vi "Write I64.vi"(8 "error in (no error)":errorcluster, 9 "Timeout (ms)":i32, 10 "Data":i64, 11 "CIFTag in":refnum<class "CIF_CIPC_Chn_I64.lvclass">) -> (0 "error out":errorcluster, 1 "timed out?":bool, 3 "CIFTag out":refnum<class "CIF_CIPC_Chn_I64.lvclass">)   [LabVIEW 2021, in "CIF_CIPC_Chn_I64.lvclass"]
uses:
  CIF_CIPC_Chn_I64.lvclass
  D:/dev/Packages/CIF_Channels_Core/src/CIFChannels/CIFChannels.lvclass
  D:/dev/Packages/CIF_Channels_Core/src/CIPC_Channels/CIF_CIPC_Chan/CIF_CIPC_Chn.lvclass
  CIFChannels/CIFChannels.lvclass/CIFChannels.ctl
  CIF_CIPC_Chan/CIF_CIPC_Chn.lvclass/CIF_CIPC_Chn.ctl
  CIF_CIPC_Chn_I64.lvclass/CIF_CIPC_Chn_I64.ctl
  CIF_CIPC_Chan/Accessors/Read CIPC Channel.vi
  Write I64 Direct.vi/4dec1408-e4ff-48ac-a735-b713bf84484a.vi
  CIFChannels/Accessors/Read Tag Forced.vi
  <vilib>/CIF Foundation/CIF CIPC/SubVIs/Check Error.vi
  <vilib>/CIF Foundation/CIF CIPC/SubVIs/Get Element Write Position.vi
  <vilib>/CIF Foundation/CIF CIPC/SubVIs/Notify Of New Write.vi
  <vilib>/CIF Foundation/CIF CIPC/SubVIs/Get dll Path.vi
  <vilib>/CIF Foundation/CIF CIPC/SubVIs/Get Element Info Variant.vi
  <vilib>/Utility/error.llb/Trim Whitespace.vi
  <vilib>/Utility/error.llb/Error Cluster From Error Code.vi
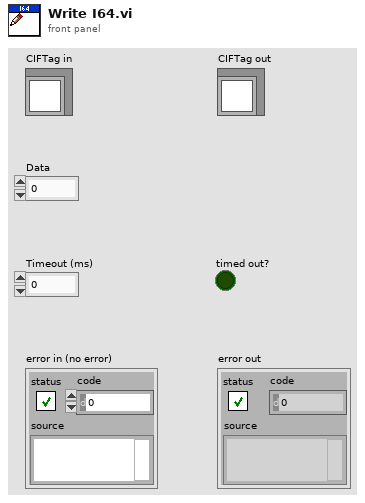
[diagram p1: front panel]
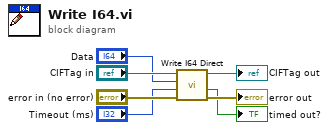
[diagram p0: block diagram]
diagram:
  n1 = call "Write I64 Direct.vi"("error in (no error)"="error in (no error)", "Timeout (ms)"="Timeout (ms)", "Data"="Data", "CIFTag in"="CIFTag in") -> ("error out"=→"error out":errorcluster, "timed out?"=→"timed out?":bool, "CIFTag out"=→"CIFTag out":refnum<class "CIF_CIPC_Chn_I64.lvclass">)  [unwired: 5 in]
